vi "FeedbackDecode_CombineMSMSPackets.vi"(1 "SphereArray":dbl[][](array[numeric])=[[0.0, 0.0, 0.1, 0.0, 1.0], [0.0, 0.0, 0.1, 0.0, 1.0], [0.0, 0.0, 0.1, 0.0, 1.0], [0.0, 0.0, 0.1, 0.0, 1.0], [0.0, 0.0, 0.1, 0.0, 1.0], [0.0, 0.0, 0.1, 0.0, 1.0]] min=-1.0 max=1.0, 2 "MvntArray":dbl[](array[numeric])=[0.0, 0.0, 0.0, 0.0, 0.0, 0.0, 0.0, 0.0, 0.0, 0.0, 0.0] min=-1.0 max=1.0) -> ()   [LabVIEW 2020]
panel:
  # "Thumb"
  # "Thumb"
  # "Index"
  # "Index"
  # "Middle"
  # "Middle"
  # "Ring"
  # "Ring"
  # "Little"
  # "Little"
  # "Wrist"
  # "ThumbInt"
  # "PosFlex"
  # "PosInt"
  # "Radius"
  # "Color"
  # "Vis"
  # "IndexInt"
  # "Ring Int"
  # "WristPitch"
  # "WristYaw"
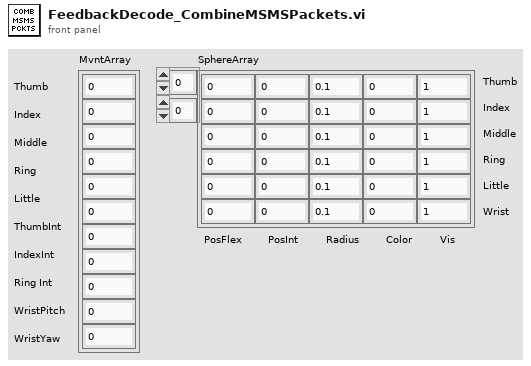
[diagram p1: front panel]
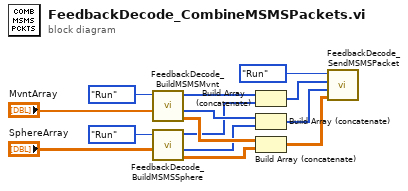
[diagram p0: block diagram]
diagram:
  n1 = call "FeedbackDecode_BuildMSMSMvnt.vi"("MvntArray"="MvntArray", "Mode"=enum16{"Initialize", "Run"}."Run") -> ("CompVals"=w10:sgl[][], "FNums"=w8:i16[], "CompIdxs"=w6:i32[])  [unwired: 5 in]
  n2 = call "FeedbackDecode_BuildMSMSSphere.vi"("SphereArray"="SphereArray", "Mode"=enum16{"Initialize", "Run"}."Run") -> ("CompVals"=w11:sgl[][], "FNums"=w9:i16[], "CompIdxs"=w7:i32[])  [unwired: 5 in]
  n3 = Build Array (concatenate)(w6, w7) -> (w12:i32[])
  n4 = Build Array (concatenate)(w8, w9) -> (w13:i16[])
  n5 = Build Array (concatenate)(w10, w11) -> (w14:sgl[][])
  n6 = call "FeedbackDecode_SendMSMSPacket.vi"("CompVal"=w14, "FNum"=w13, "CompIdx"=w12, "Mode"=enum16{"Initialize", "Run", "Close"}."Run") -> ()  [unwired: 3 in]
